vi "HeaterNVMonitor.vi"   [LabVIEW 2016]
uses:
  Instrument_Setup.vi
  Global/Global Variables/Data_Display_global.vi
types:
  T1 = typedef "ITCIO.ctl" = cluster{"Address":T2, "Version":T3, "Ch 1 dec places":i16, "Ch 2 dec places":i16, "Ch 3 dec places":i16, "Ch1 Name":string, "Ch2 Name":string, "Ch3 Name":string}
  T2 = typedef "OxfordAddress.ctl" = cluster{"Com Port":i32, "ISOBUS Address":i32, "GPIB Address":i16, "Communication":enum16{"RS232", "ISOBUS", "GPIB", "Gateway"}}
  T3 = typedef "ITCVersion.ctl" = enum16{"ITC502", "ITC503", "ITC601"}
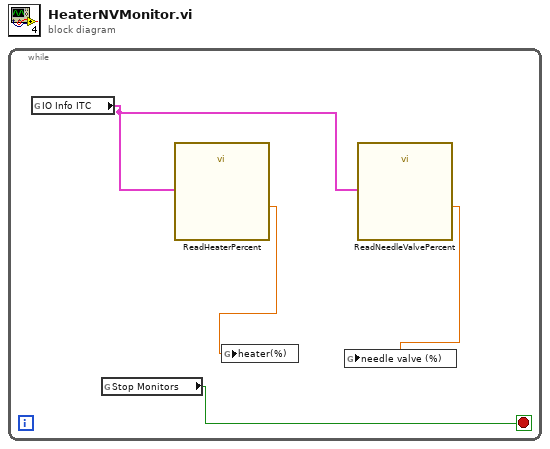
[diagram p0: block diagram]
diagram:
  n1 = while {
    stop <- w1 stop-if-true
    n2 = global read "Instrument_Setup.vi" "IO Info ITC"() -> (w2:T1)
    n3 = global read "Data_Display_global.vi" "Stop Monitors"() -> (w1:bool)
    n4 = call "ReadHeaterPercent.vi"("ITC IO Info"=w2) -> ("Actual heater  %"=w4:dbl)  [unwired: 1 in, 1 out]
    n5 = global write "Data_Display_global.vi" "heater(%)"(w4) -> ()
    n6 = call "ReadNeedleValvePercent.vi"("IO Info"=w2) -> ("Actual Needle Valve  %"=w3:dbl)  [unwired: 1 in, 1 out]
    n7 = global write "Data_Display_global.vi" "needle valve (%)"(w3) -> ()
  }
